vi "getProtocolLevel.vi"(11 "CONNECT in":refnum<class "CONNECT.lvclass">) -> (2 "Protocol Level":u8 format="%08b", 3 "CONNECT out":refnum<class "CONNECT.lvclass">)   [LabVIEW 2013, in "MQTT_Control_Packets.lvlib" / "CONNECT.lvclass"]
uses:
  CONNECT.lvclass
  ControlPacket/ControlPacket.lvclass/ControlPacket.ctl
  MQTT_311/MQTTVersion.lvclass
  ControlPacket/ControlPacket.lvclass
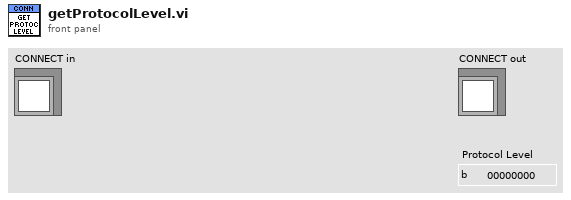
[diagram p1: front panel]
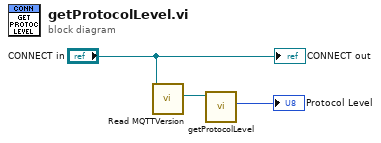
[diagram p0: block diagram]
diagram:
  n1 = call "Read MQTTVersion.vi"("ControlPacket in"="CONNECT in") -> ("MQTTVersion"=w2:refnum<class "MQTTVersion.lvclass">)  [unwired: 9 in, 1 out]
  n2 = call-dynamic "getProtocolLevel.vi"("MQTTVersion in"=w2) -> ("Protocol Level"=→"Protocol Level":u8)  [unwired: 9 in, 1 out]
  "CONNECT out" <- "CONNECT in"
